vi "GetIdentification.vi"(8 "error in (no error)":errorcluster, 11 "DigitalOutput_Simulation In":refnum<class "TesteractHAL_DigitalOutput_Simulation.lvclass">) -> (0 "error out":errorcluster, 1 "Device ID":T1, 2 "Device ID Source":T2, 3 "DigitalOutput_Simulation Out":refnum<class "TesteractHAL_DigitalOutput_Simulation.lvclass">)   [LabVIEW 2017, in "TesteractHAL_DigitalOutput_Simulation.lvlib" / "TesteractHAL_DigitalOutput_Simulation.lvclass"]
uses:
  TesteractHAL_DigitalOutput_Simulation.lvclass
  Program Files (x86)/Testeract/HWLib/HAL/Device/TesteractHAL_Device.lvlibp/DeviceIDSourceEnum.ctl
  Program Files (x86)/Testeract/HWLib/HAL/Device/TesteractHAL_Device.lvlibp/DeviceID.ctl
  Program Files (x86)/Testeract/HWLib/HAL/Device/TesteractHAL_Device.lvlibp
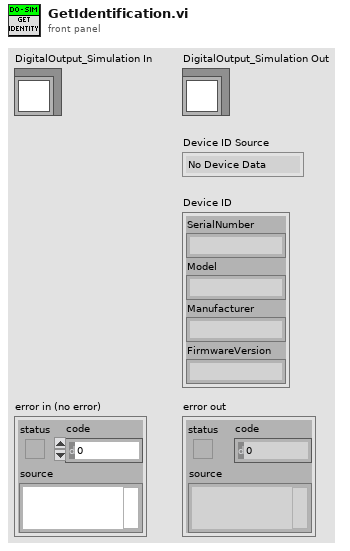
[diagram p1: front panel]
types:
  T1 = typedef "TesteractHAL_Device.lvlibp/DeviceID.ctl" = cluster{"SerialNumber":string, "Model":string, "Manufacturer":string, "FirmwareVersion":string}
  T2 = typedef "TesteractHAL_Device.lvlibp/DeviceIDSourceEnum.ctl" = enum16{"No Device Data", "From DeviceCFG", "From Hardware Device"}
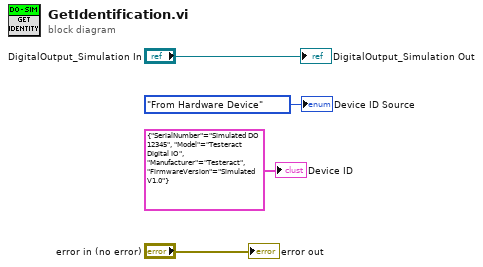
[diagram p0: block diagram]
diagram:
  "error out" <- "error in (no error)"
  "DigitalOutput_Simulation Out" <- "DigitalOutput_Simulation In"
  "Device ID Source" <- DeviceIDSourceEnum."From Hardware Device" ("Device ID Source")
  "Device ID" <- T1 {"SerialNumber"="Simulated DO 12345", "Model"="Testeract Digital IO", "Manufacturer"="Testeract", "FirmwareVersion"="Simulated V1.0"} ("Device ID")
